vi "SRV_PM_Dequeue and Parse Packet.vi"(0 "SRV_Packets queue":refnum<queue>, 11 "error in (no error)":errorcluster) -> (1 "Command Type":u8[](array[numeric]) format="%.0x", 2 "Sender":u8[](array[numeric]) format="%.0x", 3 "Timestamp":u8[](array[numeric]) format="%.0x", 4 "Packet":T1 {"Packet Data" format="%.0x"}, 6 "Data Field":u8[](array[numeric]) format="%.0x", 8 "Data String":string, 10 "Checksum":u8[](array[numeric]) format="%.0x", 13 "Data Field Length":u16 format="%.0x", 14 "Extra Bytes":u8[](array[numeric]) format="%.0x", 15 "error out":errorcluster)   [LabVIEW 2009]
uses:
  SRV_PM_Packet.ctl
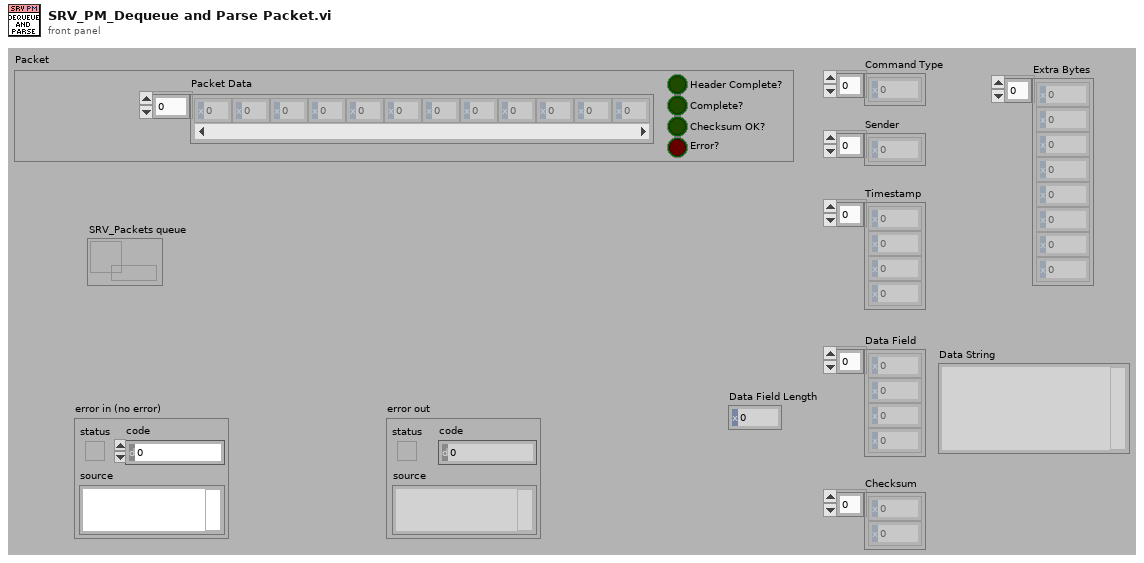
[diagram p1: front panel]
types:
  T1 = typedef "SRV_PM_Packet.ctl" = cluster{"Packet Data":u8[], "Header Complete?":bool, "Complete?":bool, "Checksum OK?":bool, "Error?":bool}
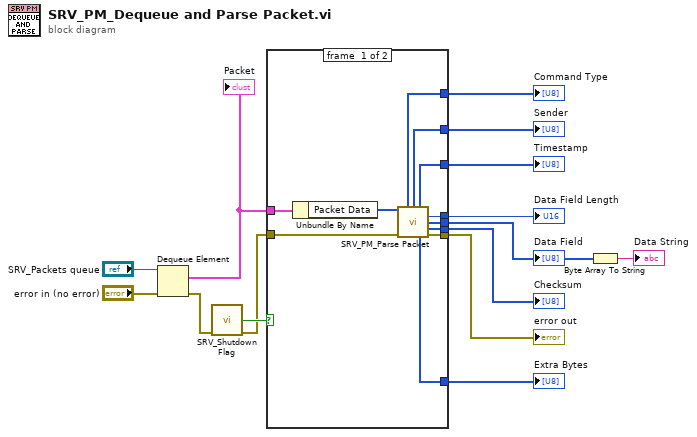
[diagram p0: block diagram]
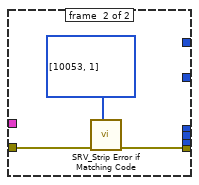
[diagram p2: hidden frame]
diagram:
  n1 = Dequeue Element(queue="SRV_Packets queue", error in (no error)="error in (no error)") -> (element=w5:T1, error out=w2:errorcluster)  [unwired: 1 in, 2 out]
  "Packet" <- w5
  n2 = call "SRV_Shutdown Flag.vi"("error in (no error)"=w2) -> ("Shutdown Flag out"=w3:bool, "error out"=w1:errorcluster)  [unwired: 13 in]
  n3 = case shown="False" w3 {
    tunnel: [w26 w27] -> w15
    tunnel: [w25 _] -> w14
    tunnel: [w24 _] -> w13
    tunnel: [w23 _] -> w12
    tunnel: [w22 _] -> w11
    tunnel: [w21 _] -> w10
    tunnel: [w20 _] -> w9
    tunnel: [w19 _] -> w7
    tunnel: w1 -> [w16 w28]
    tunnel: w5 -> [w18 _]
    frame #0 {
      n4 = Unbundle By Name(w18) -> ("Packet Data"=w17:u8[])
      n5 = call "SRV_PM_Parse Packet.vi"("Packet"=w17, "error in (no error)"=w16) -> ("Command Type"=w25:u8[], "Sender"=w24:u8[], "Timestamp"=w23:u8[], "Data Field Length"=w22:u16, "Data Field"=w19:u8[], "Checksum"=w21:u8[], "Extra Bytes"=w20:u8[], "error out"=w26:errorcluster)  [unwired: 4 in, 2 out]
    }
    frame #1 {
      n6 = call "SRV_Strip Error if Matching Code.vi"("error in (no error)"=w28, "Strip Codes"=i32[] [10053, 1]) -> ("error out"=w27:errorcluster)  [unwired: 8 in]
    }
  }
  "error out" <- w15
  "Command Type" <- w14
  "Sender" <- w13
  "Timestamp" <- w12
  "Data Field" <- w7
  "Checksum" <- w10
  "Data Field Length" <- w11
  "Extra Bytes" <- w9
  n7 = Byte Array To String(unsigned byte array=w7) -> (string=→"Data String":string)
